vi "Main.vi"(10 "RQMHStartup":refnum<class "RQMHStartup.lvclass">, 11 "ModuleManager in":refnum<class "ModuleManager.lvclass">) -> ()   [LabVIEW 2024, in "ModuleManager.lvclass"]
uses:
  ModuleManager.lvclass
  RQMHCore/Startup/RQMHStartup.lvclass
  RQMHCore/ModQueue/RQMHMessageQueue.lvclass/RQMHMessageQueue.ctl
  RQMHCore/DebugTrace/DebugTraceHandle/StartArgs.ctl
  RQMHCore/ModuleCore/InitialiseReplyArgs.ctl
  <vilib>/Utility/miscctls.llb/LVPointTypeDef.ctl
  RQMHCore/ModuleCore/RQMHModule.lvclass/RQMHModule.ctl
  Do Something ReplyArgs.ctl
  Do Something Args.ctl
  RQMHCore/ModQueue/Delacor_lib_QMH_Enqueue Message (Array).vi
  RQMHCore/ModuleCore/Read ModuleName.vi
  RQMHCore/ModuleCore/Read External Start.vi
  RQMHCore/ModQueue/RQMHMessageQueue.lvclass
  RQMHCore/ModuleCore/RQMHModule.lvclass
  RQMHCore/Shared/RQMHShared.lvlib
  RQMHCore/DebugTrace/FGVWithEventTrace/FGVWithEventTrace.lvclass
  RQMHCore/DebugTrace/DebugTraceHandle/DebugTraceHandle.lvclass
panel:
  in  "Update":bool
  in  "Module Tree":string(tree)
  out "error out":errorcluster
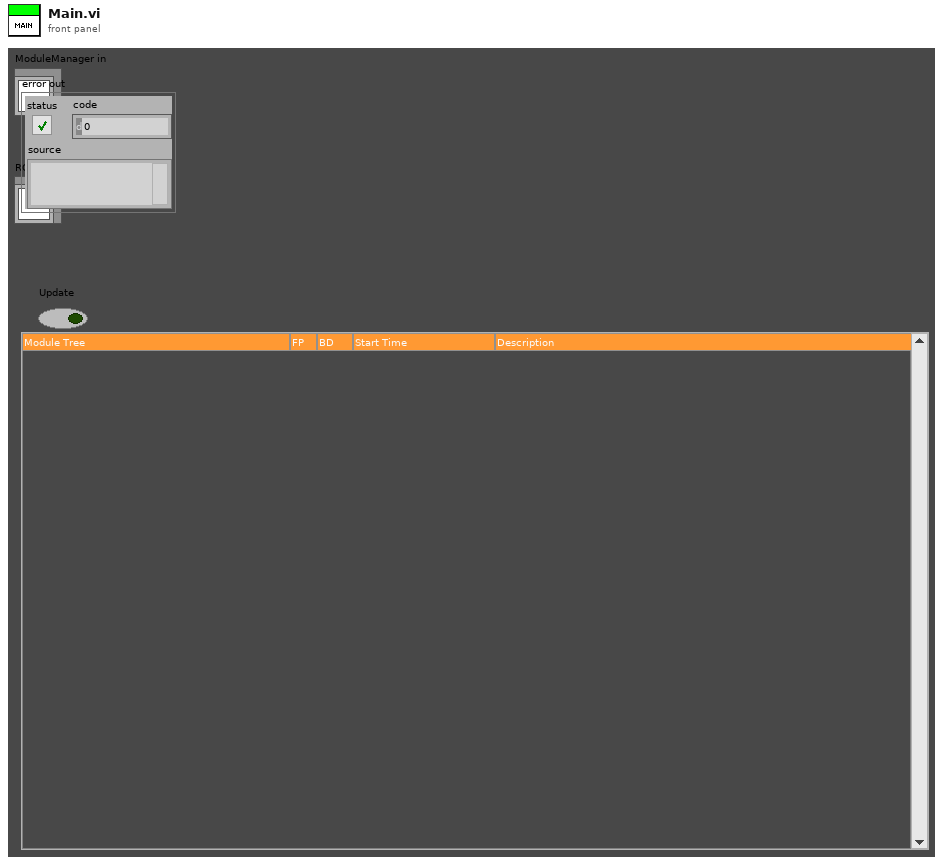
[diagram p1: front panel]
types:
  T1 = typedef "ModuleManager.lvclass/Request Events--cluster.ctl" = cluster{"Do Something":refnum<user-event>}
  T2 = cluster{"Stop Module":refnum<user-event>, "Requests":T1}
  T3 = cluster{"Module Tree":refnum<vi>, "Update UI":bool}
  T4 = typedef "DebugTraceHandle.lvclass/StartArgs.ctl" = cluster{"Caller":string, "This":string, "Alias":string, "StartTime":timestamp}
  T5 = typedef "LVPointTypeDef.ctl" = cluster{"Horizontal":i16, "Vertical":i16}
  T6 = enum32{"Invalid", "Standard", "Closed", "Hidden", "Minimized", "Maximized"}
  T7 = typedef "RQMHModule.lvclass/InitialiseReplyArgs.ctl" = cluster{"Did Init?":bool}
  T8 = typedef "ModuleManager.lvclass/Do Something Args.ctl" = cluster{"Msg":string}
  T9 = typedef "ModuleManager.lvclass/Do Something ReplyArgs.ctl" = cluster{"Value":dbl, "Boolean":bool}
  T10 = typedef "RQMHModule.lvclass/Reply.ctl" = cluster{"Expects Reply":bool, "Reply":refnum<notifier>}
  T11 = typedef "LVPoint32TypeDef.ctl" = cluster{"Horizontal":i32, "Vertical":i32}
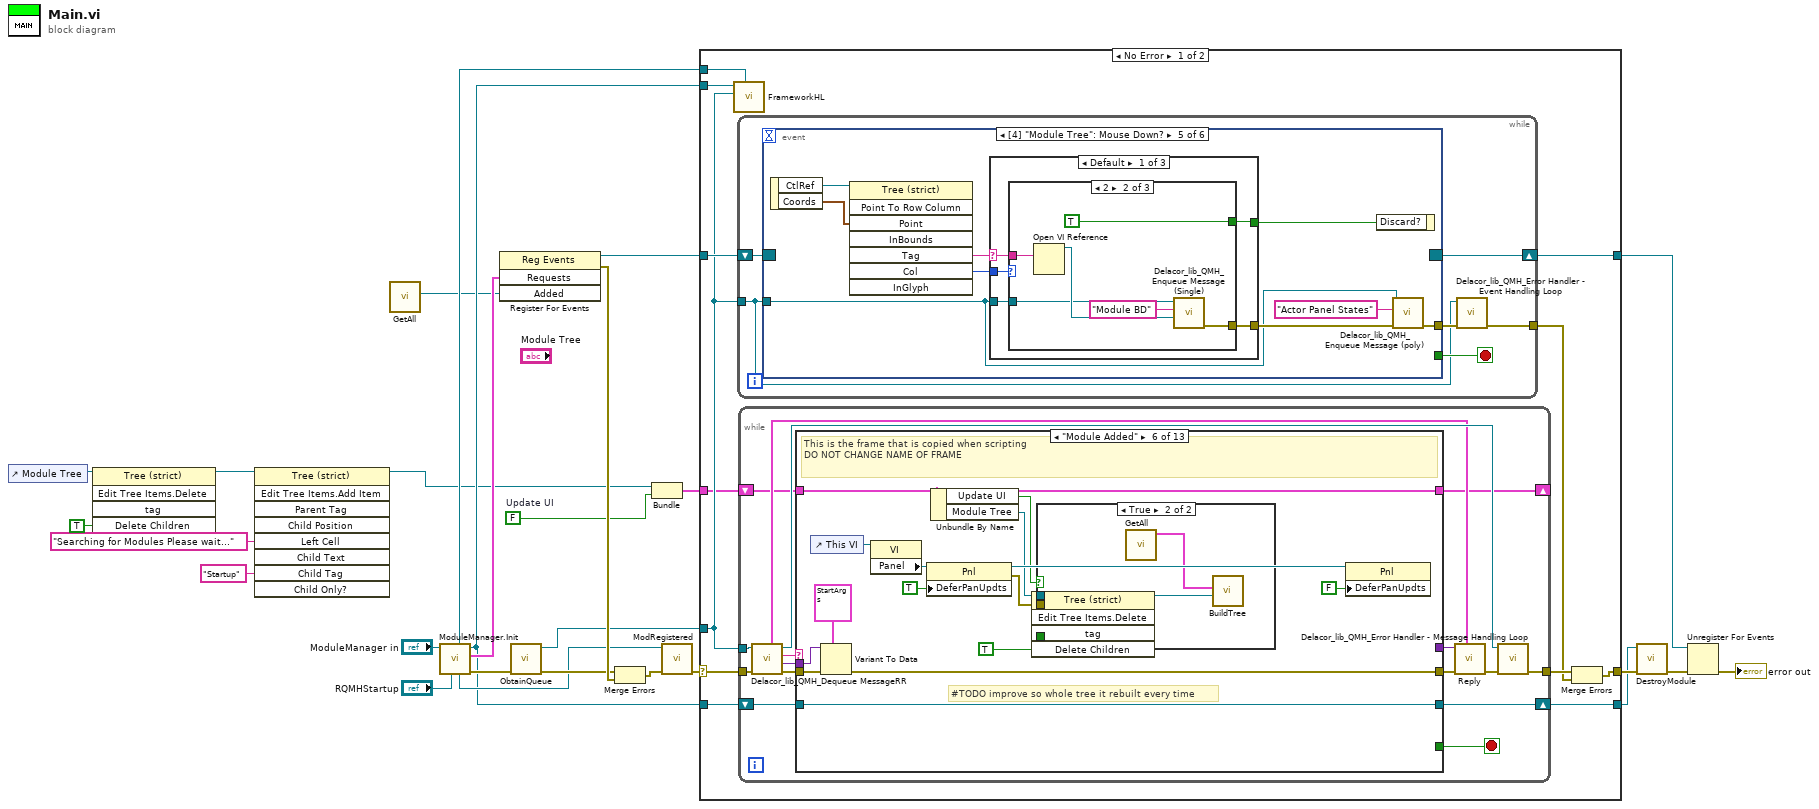
[diagram p0: block diagram]
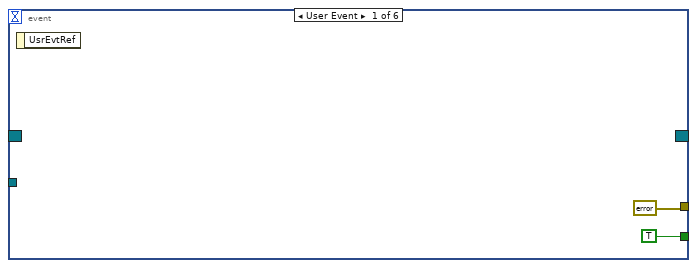
[diagram p2: hidden frame]
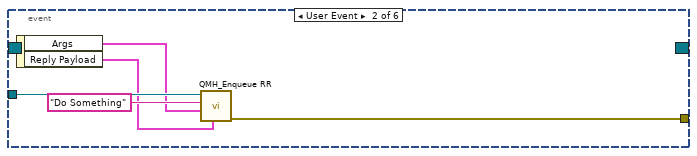
[diagram p3: hidden frame]
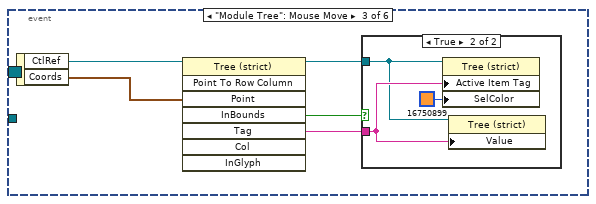
[diagram p4: hidden frame]
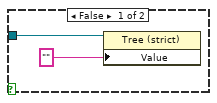
[diagram p5: hidden frame]
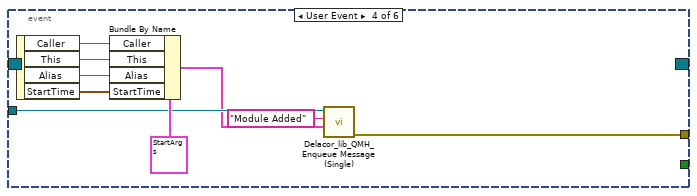
[diagram p6: hidden frame]
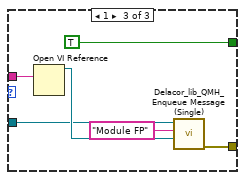
[diagram p8: hidden frame]
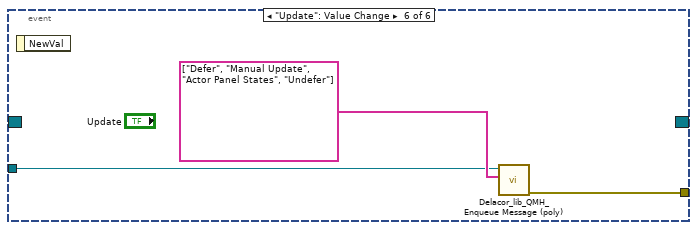
[diagram p11: hidden frame]
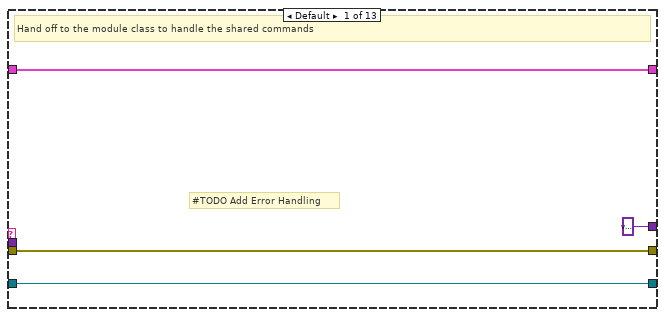
[diagram p12: hidden frame]
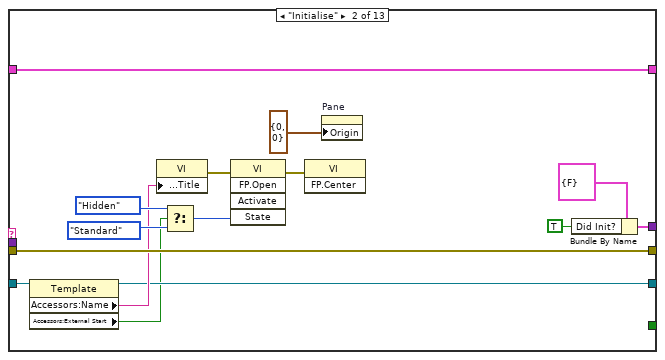
[diagram p13: hidden frame]
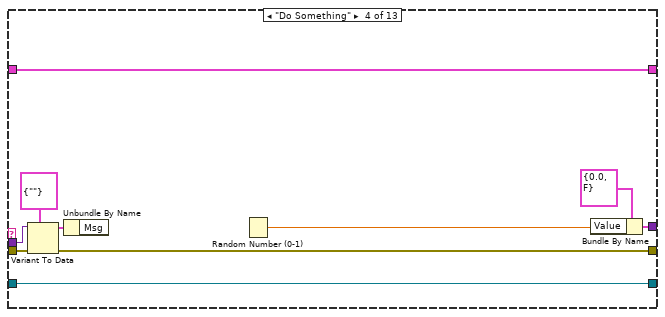
[diagram p15: hidden frame]
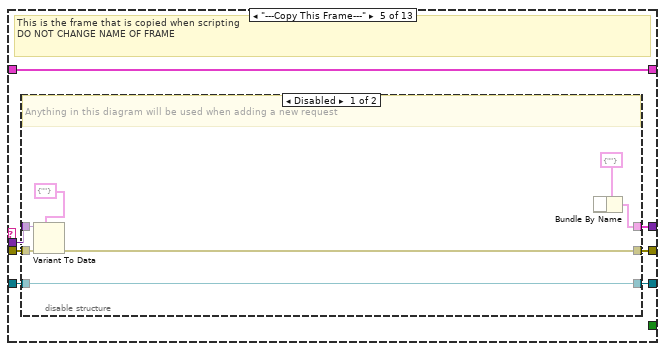
[diagram p16: hidden frame]
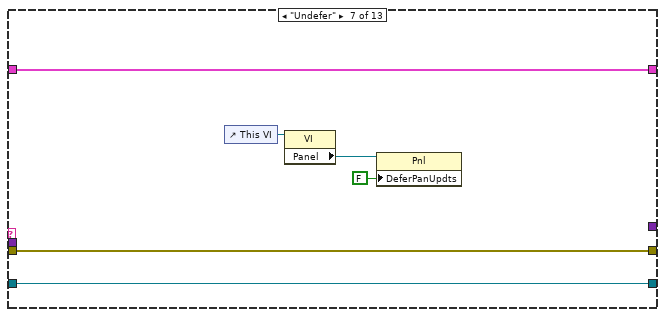
[diagram p19: hidden frame]
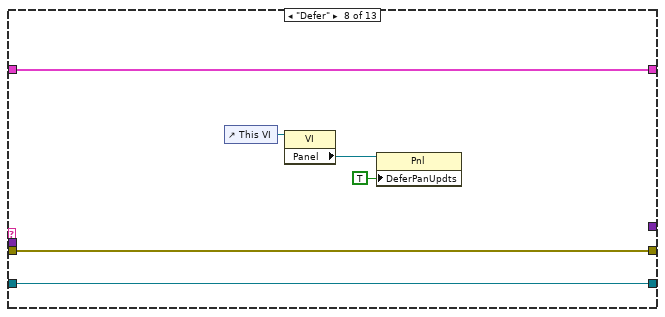
[diagram p20: hidden frame]
diagram:
  w7 = FALSE  # Update UI
  n1 = control-ref of="Module Tree"() -> (w4:refnum<vi>)
  n2 = invoke class="Tree (strict)" method="Edit Tree Items.Delete"(reference=w4, "Delete Children"=TRUE ("Delete Children?")) -> (reference out=w2:refnum<vi>)  [unwired: 3 in, 4 out]
  n3 = invoke on="Invoke Node" class="Tree (strict)" method="Edit Tree Items.Add Item"(reference=w2, "Left Cell"="Searching for Modules Please wait..." ("Left Cell String"), "Child Tag"="Startup") -> (reference out=w3:refnum<vi>)  [unwired: 6 in, 8 out]
  n4 = call "GetAll.vi"() -> ("Added"=w8:refnum<user-event>)  [unwired: 10 in, 1 out]
  n5 = call "ModuleManager.Init.vi"("JQMHStartup in"="RQMHStartup", "NewTemplate in"="ModuleManager in") -> ("error out"=w20:errorcluster, "Requests"=w11:T2, "NewTemplate out"=w10:refnum<class "ModuleManager.lvclass">, "JQMHStartup out"=w18:refnum<class "RQMHStartup.lvclass">, "StandardRequests"=w14:refnum<event-registration>)  [unwired: 4 in, 1 out]
  n6 = register-events(w11, w8) -> (reference out=w13:refnum<event-registration>, error out=w27:errorcluster)  [unwired: 2 in]
  n7 = call "ObtainQueue.vi"("error in"=w20) -> ("error out"=w19:errorcluster, "Message Queue"=w15:refnum<class "RQMHMessageQueue.lvclass">)  [unwired: 9 in]
  n8 = Merge Errors(w19, w27) -> (w16:errorcluster)
  n9 = Bundle("Module Tree"=w3, "Update UI"=w7) -> (w9:T3)  [unwired: 1 in]
  n10 = call "ModRegistered.vi"("error in (no error)"=w16, "JQMHStartup in"=w18) -> ("error out"=w17:errorcluster)  [unwired: 9 in]
  n11 = case "RQMH_MAIN" shown="No Error" w17 {
    selector: w17 -> [w36 w275]
    tunnel: w10 -> [w39 w274]
    tunnel: [w38 w277] -> w26
    tunnel: w13 -> [w37 w277]
    tunnel: w15 -> [w30 w276]
    tunnel: [w35 w274] -> w12
    tunnel: [w32 w273] -> w23
    tunnel: w10 -> [w31 _]
    tunnel: w14 -> [w29 w272]
    tunnel: w9 -> [w28 _]
    frame No Error {
      n12 = call-dynamic "FrameworkHL.vi"("StandardRequests"=w29, "Message Queue"=w30, "JQMHModule in"=w31) -> ()  [unwired: 9 in]
      n13 = while {
        shift-right: [w45] -> w38
        shift-left: w37 -> [w40]
        tunnel: w30 -> [w41]
        tunnel: [w42] -> w33
        stop <- w44 stop-if-true
        n14 = event "RQMH_EVENT_MAIN" shown="[4] \"Module Tree\": Mouse Down?" {
          selector: w40 -> [_ _ _ _ _ _]
          dyn-events: [_ _ _ _ _ _] -> w45
          timeout: _ -> [_ _ _ _ _ _]
          tunnel: [TRUE _ _ _ _ _] -> w44
          tunnel: w41 -> [_ w52 _ w66 w72 w98]
          tunnel: [errorcluster {"status"=FALSE, "code"=0, "source"=""} ("error out") w49 _ w64 w74 w100] -> w43
          event User Event {
            n15 = event-data() -> ()  [unwired: 1 in, 1 out]
          }
          event User Event {
            n16 = event-data() -> ("Args"=w50:T8, "Reply Payload"=w48:T10)  [unwired: 1 in]
            n17 = call "QMH_Enqueue RR.vi"("Reply"=w48, "Message Data"=w50, "Message"="Do Something", "Message Queue in"=w52) -> ("error out"=w49:errorcluster)  [unwired: 6 in, 1 out]
          }
          event "Module Tree": Mouse Move {
            n18 = event-data() -> ("CtlRef"=w53:refnum<vi>, "Coords"=w54:T11)  [unwired: 1 in]
            n19 = invoke class="Tree (strict)" method="Point To Row Column"(reference=w53, "Point"=w54) -> (reference out=w57:refnum<vi>, "InBounds"=w55:bool, "Tag"=w56:string)  [unwired: 6 in, 5 out]
            n20 = case shown="True" w55 {
              tunnel: w57 -> [w58 w60]
              tunnel: w56 -> [_ w61]
              frame False {
                n21 = property class="Tree (strict)"(reference=w58, "Value"="") -> ()  [unwired: 1 in, 2 out]
              }
              frame True {
                n22 = property class="Tree (strict)"(reference=w60, "Active Item Tag"=w61, "SelColor"=u32 16750899 ("Selection Color")) -> ()  [unwired: 1 in, 2 out]
                n23 = property class="Tree (strict)"(reference=w60, "Value"=w61) -> ()  [unwired: 1 in, 2 out]
              }
            }
          }
          event User Event {
            n24 = event-data() -> ("Caller"=w70:string, "This"=w69:string, "Alias"=w68:string, "StartTime"=w67:timestamp)  [unwired: 1 in]
            n25 = Bundle By Name(cluster=T4 {"Caller"="", "This"="", "Alias"="", "StartTime"=timestamp(0 s since 1904-01-01)} ("StartArgs"), "Caller"=w70, "This"=w69, "Alias"=w68, "StartTime"=w67) -> (w65:T4)
            n26 = call "Delacor_lib_QMH_Enqueue Message (Single).vi"("Message Data"=w65, "Message"="Module Added", "Message Queue in"=w66) -> ("error out"=w64:errorcluster)  [unwired: 7 in, 1 out]
          }
          event "Module Tree": Mouse Down? {
            n27 = event-data() -> ("CtlRef"=w80:refnum<vi>, "Coords"=w79:T11)  [unwired: 1 in]
            n28 = invoke class="Tree (strict)" method="Point To Row Column"(reference=w80, "Point"=w79) -> ("Tag"=w77:string, "Col"=w78:i32)  [unwired: 6 in, 6 out]
            n29 = case shown="Default" w77 {
              selector: w77 -> [w81 _ _]
              tunnel: w78 -> [w85 _ _]
              tunnel: w72 -> [w83 _ _]
              tunnel: [w84 _ _] -> w76
              tunnel: [w82 _ _] -> w75
              frame Default {
                n30 = case shown="2" w85 {
                  tunnel: [_ TRUE TRUE] -> w84
                  tunnel: w83 -> [_ w88 w94]
                  tunnel: [_ w87 w93] -> w82
                  tunnel: w81 -> [_ w86 w92]
                  frame Default {
                  }
                  frame 2 {
                    n31 = Open VI Reference(vi path=w86) -> (vi reference=w90:refnum<vi>)  [unwired: 5 in, 1 out]
                    n32 = call "Delacor_lib_QMH_Enqueue Message (Single).vi"("Message Data"=w90, "Message"="Module BD", "Message Queue in"=w88) -> ("error out"=w87:errorcluster)  [unwired: 7 in, 1 out]
                  }
                  frame 1 {
                    n33 = Open VI Reference(vi path=w92) -> (vi reference=w96:refnum<vi>)  [unwired: 5 in, 1 out]
                    n34 = call "Delacor_lib_QMH_Enqueue Message (Single).vi"("Message Data"=w96, "Message"="Module FP", "Message Queue in"=w94) -> ("error out"=w93:errorcluster)  [unwired: 7 in, 1 out]
                  }
                }
              }
              frame "TREE_COLUMN_HEADERS" {
              }
              frame "Startup" {
              }
            }
            n35 = event-data("Discard?"=w76) -> ()  [unwired: 1 in, 1 out]
            n36 = call-poly "Delacor_lib_QMH_Enqueue Message (poly).vi"("error in"=w75, "Message"="Actor Panel States", "Message Queue in"=w72) -> ("error out"=w74:errorcluster)  [unwired: 7 in, 1 out]
          }
          event "Update": Value Change {
            n37 = event-data() -> ()  [unwired: 1 in, 1 out]
            n38 = call-poly "Delacor_lib_QMH_Enqueue Message (poly).vi"("Message Array"=string[] ["Defer", "Manual Update", "Actor Panel States", "Undefer"] ("Message"), "Message Queue in"=w98) -> ("error out"=w100:errorcluster)  [unwired: 8 in, 1 out]
          }
        }
        n39 = call-dynamic "Delacor_lib_QMH_Error Handler - Event Handling Loop.vi"("error in"=w43, "Message Queue in"=w41) -> ("dup error in"=w42:errorcluster)  [unwired: 8 in, 1 out]
      }
      n40 = while {
        tunnel: w30 -> [w111]
        tunnel: w36 -> [w110]
        shift-right: [w113] -> w35
        shift-left: w39 -> [w114]
        tunnel: [w112] -> w34
        shift-right: [w101] -> _
        shift-left: w28 -> [w102]
        stop <- w116 stop-if-true
        n41 = call-dynamic "Delacor_lib_QMH_Dequeue MessageRR.vi"("error in"=w110, "Message Queue in"=w111) -> ("error out"=w109:errorcluster, "Message Data"=w107:variant, "Message"=w108:string, "Message Queue out"=w115:refnum<class "RQMHMessageQueue.lvclass">, "Reply"=w103:T10)  [unwired: 5 in]
        n42 = case "RQMH_MESSAGE_CASES" shown="\"Module Added\"" w108 {
          tunnel: [_ _ _ _ _ _ _ _ _ _ _ _ TRUE] -> w116
          tunnel: w114 -> [w119 w123 w137 w148 w153 w177 w189 w195 w202 w211 w243 w266 w270]
          tunnel: w107 -> [_ _ _ w144 w151 w176 _ _ _ _ w242 w265 _]
          tunnel: w109 -> [w120 w135 w138 w143 w155 w179 w190 w196 w203 w207 w244 w267 w269]
          tunnel: [w120 w135 w138 w142 w154 w178 w190 w196 w203 w208 w232 w260 w269] -> w106
          tunnel: [w119 w124 w137 w148 w152 w177 w189 w195 w202 w211 w243 w266 w270] -> w113
          tunnel: [variant w134 _ w147 w150 _ _ _ _ _ _ _ _] -> w104
          tunnel: w102 -> [w117 w121 w136 w139 w149 w168 w188 w194 w200 w210 w241 w264 w268]
          tunnel: [w117 w121 w136 w139 w149 w168 w188 w194 w200 w210 w241 w264 w268] -> w101
          frame Default {
            # "#TODO Add Error Handling"
            # "Hand off to the module class to handle the shared commands"
          }
          frame "Initialise" {
            n43 = property class="Template"(reference=w123) -> (reference out=w124:refnum<class "ModuleManager.lvclass">, "Accessors:Name"=w125:string, "Accessors:External Start"=w122:bool)  [unwired: 1 in, 1 out]
            n44 = property on="Property Node" class="VI"("Front Panel.Title"=w125) -> (error out=w132:errorcluster)  [unwired: 2 in, 1 out]
            n45 = Select(t=T6."Hidden" ("State"), s=w122, f=T6."Standard" ("State")) -> (s? t:f=w128:T6)
            n46 = invoke on="Invoke Node" class="VI" method="FP.Open"(error in=w132, "State"=w128) -> (error out=w131:errorcluster)  [unwired: 3 in, 4 out]
            n47 = invoke on="Invoke Node" class="VI" method="FP.Center"(error in=w131) -> ()  [unwired: 2 in, 3 out]
            n48 = property on="Pane" class="Pane"("Origin"=T5 {"Horizontal"=0, "Vertical"=0}) -> ()  [unwired: 2 in, 2 out]
            n49 = Bundle By Name(cluster=T7 {"Did Init?"=FALSE} ("Args"), "Did Init?"=TRUE) -> (w134:T7)
          }
          frame "---Module Specific---" {
          }
          frame "Do Something" {
            n50 = Variant To Data(error in=w143, type=T8 {"Msg"=""} ("Do Something Args"), Variant=w144) -> (data=w140:T8, error out=w142:errorcluster)
            n51 = Unbundle By Name(w140) -> ()  [unwired: 1 out]
            n52 = Random Number (0-1)() -> (number: 0 to 1=w145:dbl)
            n53 = Bundle By Name(cluster=T9 {"Value"=0.0, "Boolean"=FALSE}, "Value"=w145) -> (w147:T9)
          }
          frame "---Copy This Frame---" {
            # "This is the frame that is copied when scripting\nDO NOT CHANGE NAME OF FRAME"
            n54 = disable-structure shown="Disabled" {
              disable-tunnel: w155 -> [w159 w164]
              disable-tunnel: [w160 w164] -> w154
              disable-tunnel: w153 -> [w162 w163]
              disable-tunnel: [w162 w163] -> w152
              disable-tunnel: w151 -> [w161 _]
              disable-tunnel: [w157 _] -> w150
              frame Disabled {
                # "Anything in this diagram will be used when adding a new request"
                n55 = Variant To Data(error in=w159, type=cluster{string} {""} ("RQMH_MHL_MSG_PL"), Variant=w161) -> (error out=w160:errorcluster)  [unwired: 1 out]
                n56 = Bundle By Name(cluster=cluster{string} {""} ("RQMH_MHL_REPLY_PL")) -> (w157:cluster{string})  [unwired: 1 in]
              }
              frame Enabled {
              }
            }
          }
          frame "Module Added" {
            # "#TODO improve so whole tree it rebuilt every time"
            # "This is the frame that is copied when scripting\nDO NOT CHANGE NAME OF FRAME"
            n57 = control-ref of="This VI"() -> (w174:refnum<vi>)
            n58 = Variant To Data(error in=w179, type=T4 {"Caller"="", "This"="", "Alias"="", "StartTime"=timestamp(0 s since 1904-01-01)} ("StartArgs"), Variant=w176) -> (error out=w178:errorcluster)  [unwired: 1 out]
            n59 = property class="VI"(reference=w174) -> ("Panel"=w173:refnum<vi>)  [unwired: 1 in, 2 out]
            n60 = property class="Pnl"(reference=w173, "DeferPanUpdts"=TRUE ("Defer Panel Updates")) -> (reference out=w170:refnum<vi>, error out=w166:errorcluster)  [unwired: 1 in]
            n61 = Unbundle By Name(w168) -> ("Update UI"=w165:bool, "Module Tree"=w167:refnum<vi>)
            n62 = case shown="True" w165 {
              tunnel: TRUE ("Delete Children?") -> [_ w184]
              tunnel: w167 -> [_ w183]
              tunnel: w166 -> [_ w182]
              frame False {
              }
              frame True {
                n63 = invoke on="Invoke Node" class="Tree (strict)" method="Edit Tree Items.Delete"(reference=w183, error in=w182, "Delete Children"=w184) -> (reference out=w181:refnum<vi>)  [unwired: 2 in, 4 out]
                n64 = call "GetAll.vi"() -> ("Modules"=w180:T4[])  [unwired: 10 in, 1 out]
                n65 = call "BuildTree.vi"("TreeControl in"=w181, "Array"=w180) -> ()  [unwired: 9 in, 1 out]
              }
            }
            n66 = property class="Pnl"(reference=w170, "DeferPanUpdts"=FALSE ("Defer Panel Updates")) -> ()  [unwired: 1 in, 2 out]
          }
          frame "Undefer" {
            n67 = control-ref of="This VI"() -> (w186:refnum<vi>)
            n68 = property class="VI"(reference=w186) -> ("Panel"=w187:refnum<vi>)  [unwired: 1 in, 2 out]
            n69 = property class="Pnl"(reference=w187, "DeferPanUpdts"=FALSE ("Defer Panel Updates")) -> ()  [unwired: 1 in, 2 out]
          }
          frame "Defer" {
            n70 = control-ref of="This VI"() -> (w192:refnum<vi>)
            n71 = property class="VI"(reference=w192) -> ("Panel"=w193:refnum<vi>)  [unwired: 1 in, 2 out]
            n72 = property class="Pnl"(reference=w193, "DeferPanUpdts"=TRUE ("Defer Panel Updates")) -> ()  [unwired: 1 in, 2 out]
          }
          frame "Manual Update" {
            # "Bodge while tree rebuilding when added"
            # "This is the frame that is copied when scripting\nDO NOT CHANGE NAME OF FRAME"
            n73 = Unbundle By Name(w200) -> ("Module Tree"=w199:refnum<vi>)
            n74 = invoke on="Invoke Node" class="Tree (strict)" method="Edit Tree Items.Delete"(reference=w199, "Delete Children"=TRUE ("Delete Children?")) -> (reference out=w198:refnum<vi>)  [unwired: 3 in, 4 out]
            n75 = call "GetAll.vi"() -> ("Modules"=w197:T4[])  [unwired: 10 in, 1 out]
            n76 = call "BuildTree.vi"("TreeControl in"=w198, "Array"=w197) -> ()  [unwired: 9 in, 1 out]
          }
          frame "Actor Panel States" {
            n77 = Unbundle By Name(w210) -> ("Module Tree"=w209:refnum<vi>)
            n78 = property class="Tree (strict)"(reference=w209, error in=w207) -> (reference out=w204:refnum<vi>, error out=w208:errorcluster, "All Tags"=w206:string[])
            n79 = for {
              tunnel: w206 -> [w213] mode=indexing
              tunnel: [w223] -> w205 mode=indexing
              tunnel: w204 -> [w212]
              n80 = Open VI Reference(vi path=w213) -> (vi reference=w224:refnum<vi>, error out=w225:errorcluster)  [unwired: 5 in]
              n81 = call "FPOpen.vi"("VI in"=w224) -> ("Open?"=w219:bool)  [unwired: 8 in, 2 out]
              n82 = property class="VI"(reference=w224, error in=w225) -> (reference out=w223:refnum<vi>, error out=w215:errorcluster, "BDWin.Open"=w216:bool)
              n83 = Select(t="O", s=w219, f="X") -> (s? t:f=w220:string)
              n84 = Select(t="O", s=w216, f="X") -> (s? t:f=w214:string)
              n85 = case shown="No Error" w215 {
                tunnel: w212 -> [w231 _]
                tunnel: w213 -> [w230 _]
                tunnel: w220 -> [w228 _]
                tunnel: w214 -> [w226 _]
                frame No Error {
                  n86 = property class="Tree (strict)"(reference=w231, "Active Item Tag"=w230, "ActiveColNum"=1 ("Active Cell:Active Column Number"), "Cell String"=w228, "ActiveColNum"=2 ("Active Cell:Active Column Number"), "Cell String"=w226) -> ()  [unwired: 1 in, 2 out]
                }
                frame Error {
                }
              }
            }
            n87 = Close Reference(reference=w205) -> ()  [unwired: 1 in, 1 out]
          }
          frame "Module FP" {
            # "Toggle FP State of Module"
            n88 = Variant To Data(error in=w244, type=refnum<vi> refnum ("vi reference"), Variant=w242) -> (data=w237:refnum<vi>, error out=w238:errorcluster)
            n89 = property class="VI"(reference=w237, error in=w238) -> (reference out=w236:refnum<vi>, error out=w233:errorcluster, "FP.State"=w239:T6)
            n90 = case shown="\"Closed\", \"Hidden\"" w239 {
              tunnel: w236 -> [w248 w252]
              tunnel: [w247 w253] -> w235
              tunnel: [w245 w250] -> w234
              tunnel: w233 -> [w246 w249]
              frame "Closed", "Hidden" {
                n91 = invoke class="VI" method="FP.Open"(reference=w248, error in=w246) -> (reference out=w247:refnum<vi>, error out=w245:errorcluster)  [unwired: 3 in, 3 out]
              }
              frame Default {
                n92 = invoke class="VI" method="FP.Open"(reference=w252, error in=w249, "State"=T6."Hidden") -> (reference out=w253:refnum<vi>, error out=w250:errorcluster)  [unwired: 2 in, 3 out]
              }
            }
            n93 = Close Reference(reference=w235, error in (no error)=w234) -> (error out=w232:errorcluster)
          }
          frame "Module BD" {
            # "Toggle FP State of Module"
            n94 = Variant To Data(error in=w267, type=refnum<vi> refnum ("vi reference"), Variant=w265) -> (data=w261:refnum<vi>, error out=w262:errorcluster)
            n95 = property class="VI"(reference=w261, error in=w262) -> (reference out=w257:refnum<vi>, error out=w254:errorcluster, "BDWin.Open"=w259:bool)
            n96 = Not(x=w259) -> (.not. x?=w258:bool)
            n97 = property class="VI"(reference=w257, error in=w254, "BDWin.Open"=w258) -> (reference out=w256:refnum<vi>, error out=w255:errorcluster)
            n98 = Close Reference(reference=w256, error in (no error)=w255) -> (error out=w260:errorcluster)
          }
          frame "Exit" {
            # "Clean up and send message to EHL"
          }
        }
        n99 = call "Reply.vi"("Reply"=w103, "error in (no error)"=w106, "ReplyPayload"=w104) -> ("error out"=w105:errorcluster)  [unwired: 8 in]
        n100 = call-dynamic "Delacor_lib_QMH_Error Handler - Message Handling Loop.vi"("error in"=w105, "Message Queue in"=w115) -> ("dup error in"=w112:errorcluster)  [unwired: 8 in, 1 out]
      }
      n101 = Merge Errors(w34, w33) -> (w32:errorcluster)
    }
    frame Error {
      n102 = call-dynamic "Delacor_lib_QMH_Release Message Queue.vi"("error in"=w275, "Message Queue"=w276) -> ("error out"=w273:errorcluster)  [unwired: 9 in]
      n103 = Unregister For Events(event registration refnum=w272) -> ()  [unwired: 1 in, 1 out]
    }
  }
  n104 = call "DestroyModule.vi"("error in (no error)"=w23, "JQMHModule in"=w12) -> ("error out"=w25:errorcluster)  [unwired: 9 in]
  n105 = Unregister For Events(event registration refnum=w26, error in=w25) -> (error out=→"error out":errorcluster)
